vi "Set Default.vi"(8 "error in (no error)":errorcluster, 10 "Node":refnum<class "TreeNode.lvclass">, 11 "Tree in":refnum<class "Tree.lvclass">) -> (0 "error out":errorcluster, 2 "Node out":refnum<class "TreeNode.lvclass">, 3 "Tree out":refnum<class "Tree.lvclass">)   [LabVIEW 2012, in "MDSplus.lvlib" / "Tree.lvclass"]
doc: "Set the default position in the tree."
uses:
  <vilib>/MDSplus/Classes/Tree_Class/Tree.lvclass
  <vilib>/MDSplus/Classes/Data_Class/TreeNode_Class/TreeNode.lvclass
  <vilib>/MDSplus/Classes/Data_Class/Data.lvclass
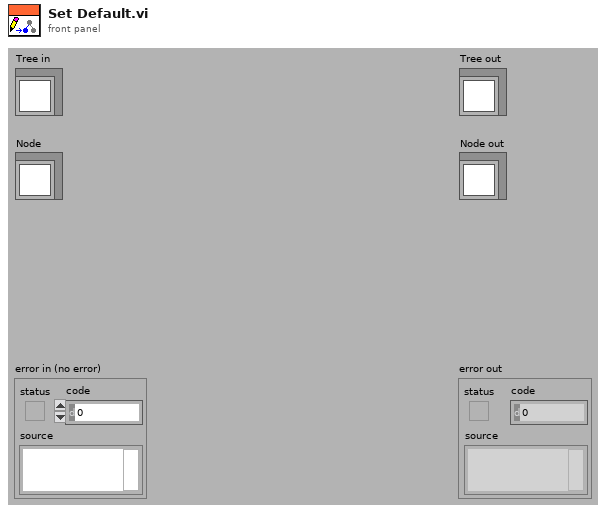
[diagram p1: front panel]
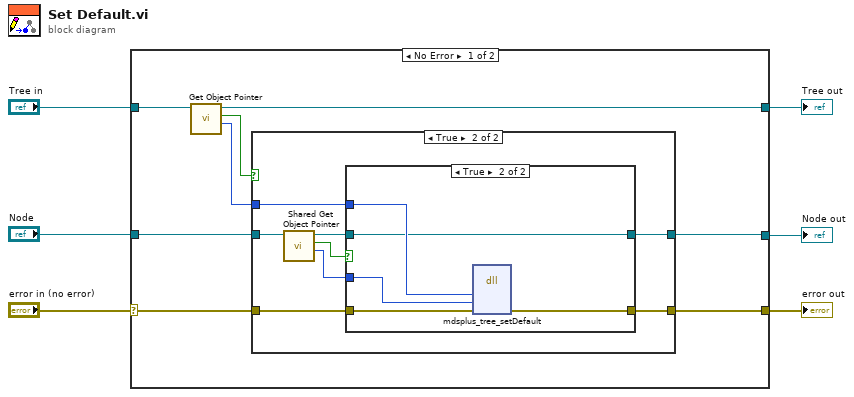
[diagram p0: block diagram]
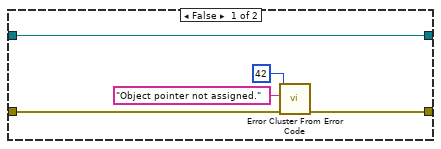
[diagram p2: hidden frame]
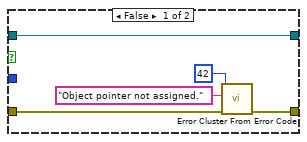
[diagram p3: hidden frame]
diagram:
  n1 = case shown="No Error" "error in (no error)" {
    selector: "error in (no error)" -> [w10 w38]
    tunnel: [w9 w38] -> w5
    tunnel: [w8 w40] -> w3
    tunnel: "Tree in" -> [w14 w40]
    tunnel: "Node" -> [w13 w39]
    tunnel: [w7 w39] -> w1
    frame No Error {
      n2 = call-dynamic "Get Object Pointer.vi"("Tree in"=w14) -> ("Object Pointer"=w11:i64, "Assigned object pointer?"=w12:bool, "Tree out"=w8:refnum<class "Tree.lvclass">)  [unwired: 8 in]
      n3 = case shown="True" w12 {
        tunnel: w13 -> [w16 w27]
        tunnel: w11 -> [_ w24]
        tunnel: w10 -> [w15 w23]
        tunnel: [w17 w22] -> w9
        tunnel: [w16 w20] -> w7
        frame False {
          n4 = call <vilib>:"Error Cluster From Error Code.vi"("error in (no error)"=w15, "error message (\"\")"="Object pointer not assigned." ("error message (\"\")"), "error code (0)"=42) -> ("error out"=w17:errorcluster)  [unwired: 6 in]
        }
        frame True {
          n5 = call <vilib>:"Shared Get Object Pointer.vi"("Data in"=w27) -> ("Object Pointer"=w25:i64, "Assigned object pointer?"=w26:bool, "Data out"=w21:refnum<class "TreeNode.lvclass">)  [unwired: 8 in]
          n6 = case shown="True" w26 {
            tunnel: w25 -> [_ w36]
            tunnel: w24 -> [_ w37]
            tunnel: w23 -> [w30 w35]
            tunnel: [w29 w33] -> w22
            tunnel: w21 -> [w28 w34]
            tunnel: [w28 w34] -> w20
            frame False {
              n7 = call <vilib>:"Error Cluster From Error Code.vi"("error in (no error)"=w30, "error message (\"\")"="Object pointer not assigned." ("error message (\"\")"), "error code (0)"=42) -> ("error out"=w29:errorcluster)  [unwired: 6 in]
            }
            frame True {
              n8 = dll-call lib="MDSobjectsLVShr" fn="mdsplus_tree_setDefault"("lvTreePtr"=w37, "lvTreeNodePtrIn"=w36, "error"=w35) -> ("error"=w33:errorcluster)  [unwired: 6 in, 2 out]
            }
          }
        }
      }
    }
    frame Error {
    }
  }
  "error out" <- w5
  "Tree out" <- w3
  "Node out" <- w1
